vi "Intialise or refresh queue.vi"(2 "When did you stick it in?":dbl, 3 "Cell Settings Array":T2(array[cluster])=[{"Measure?"=TRUE, "Area (cm^2)"=0.0, "Cell Label"="", "Cell Description"="", "Time between scans (s)"=0.0, "Cell Position"=1, "Scan settings in queue"=0, "Sample holder"=4.0}, {"Measure?"=TRUE, "Area (cm^2)"=0.0, "Cell Label"="", "Cell Description"="", "Time between scans (s)"=0.0, "Cell Position"=2, "Scan settings in queue"=0, "Sample holder"=4.0}, {"Measure?"=TRUE, "Area (cm^2)"=0.0, "Cell Label"="", "Cell Description"="", "Time between scans (s)"=0.0, "Cell Position"=3, "Scan settings in queue"=0, "Sample holder"=4.0}, {"Measure?"=TRUE, "Area (cm^2)"=0.0, "Cell Label"="", "Cell Description"="", "Time between scans (s)"=0.0, "Cell Position"=4, "Scan settings in queue"=0, "Sample holder"=4.0}, {"Measure?"=TRUE, "Area (cm^2)"=0.0, "Cell Label"="", "Cell Description"="", "Time between scans (s)"=0.0, "Cell Position"=5, "Scan settings in queue"=0, "Sample holder"=4.0}, {"Measure?"=TRUE, "Area (cm^2)"=0.0, "Cell Label"="", "Cell Description"="", "Time between scans (s)"=0.0, "Cell Position"=6, "Scan settings in queue"=0, "Sample holder"=4.0}, {"Measure?"=TRUE, "Area (cm^2)"=0.0, "Cell Label"="", "Cell Description"="", "Time between scans (s)"=0.0, "Cell Position"=7, "Scan settings in queue"=0, "Sample holder"=4.0}, {"Measure?"=TRUE, "Area (cm^2)"=0.0, "Cell Label"="", "Cell Description"="", "Time between scans (s)"=0.0, "Cell Position"=8, "Scan settings in queue"=0, "Sample holder"=4.0}, {"Measure?"=TRUE, "Area (cm^2)"=0.0, "Cell Label"="", "Cell Description"="", "Time between scans (s)"=0.0, "Cell Position"=9, "Scan settings in queue"=0, "Sample holder"=4.0}, {"Measure?"=TRUE, "Area (cm^2)"=0.0, "Cell Label"="", "Cell Description"="", "Time between scans (s)"=0.0, "Cell Position"=10, "Scan settings in queue"=0, "Sample holder"=4.0}, {"Measure?"=TRUE, "Area (cm^2)"=0.0, "Cell Label"="", "Cell Description"="", "Time between scans (s)"=0.0, "Cell Position"=11, "Scan settings in queue"=0, "Sample holder"=4.0}, {"Measure?"=TRUE, "Area (cm^2)"=0.0, "Cell Label"="", "Cell Description"="", "Time between scans (s)"=0.0, "Cell Position"=12, "Scan settings in queue"=0, "Sample holder"=4.0}, {"Measure?"=TRUE, "Area (cm^2)"=0.0, "Cell Label"="", "Cell Description"="", "Time between scans (s)"=0.0, "Cell Position"=13, "Scan settings in queue"=0, "Sample holder"=4.0}, {"Measure?"=TRUE, "Area (cm^2)"=0.0, "Cell Label"="", "Cell Description"="", "Time between scans (s)"=0.0, "Cell Position"=14, "Scan settings in queue"=0, "Sample holder"=4.0}, {"Measure?"=TRUE, "Area (cm^2)"=0.0, "Cell Label"="", "Cell Description"="", "Time between scans (s)"=0.0, "Cell Position"=15, "Scan settings in queue"=0, "Sample holder"=4.0}, {"Measure?"=TRUE, "Area (cm^2)"=0.0, "Cell Label"="", "Cell Description"="", "Time between scans (s)"=0.0, "Cell Position"=16, "Scan settings in queue"=0, "Sample holder"=4.0}] {"Scan settings in queue" items=["Regular", "Inverted"]}, 4 "Queue in":T1(array[cluster]) {"Scan settings in queue" items=["Regular", "Inverted"]; "Time of the last scan (s)" format="%<%H:%M:%S>t"; "When did you stick it in?" format="%<%H:%M:%S>t"; "Time to next scan (s)" format="%<%H:%M:%S>t"; "Time in rig (s)" format="%<%H:%M:%S>t"}) -> (0 "Queue out":T1(array[cluster]) {"Scan settings in queue" items=["Regular", "Inverted"]; "Time of the last scan (s)" format="%<%H:%M:%S>t"; "When did you stick it in?" format="%<%H:%M:%S>t"; "Time to next scan (s)" format="%<%H:%M:%S>t"; "Time in rig (s)" format="%<%H:%M:%S>t"})   [LabVIEW 2011]
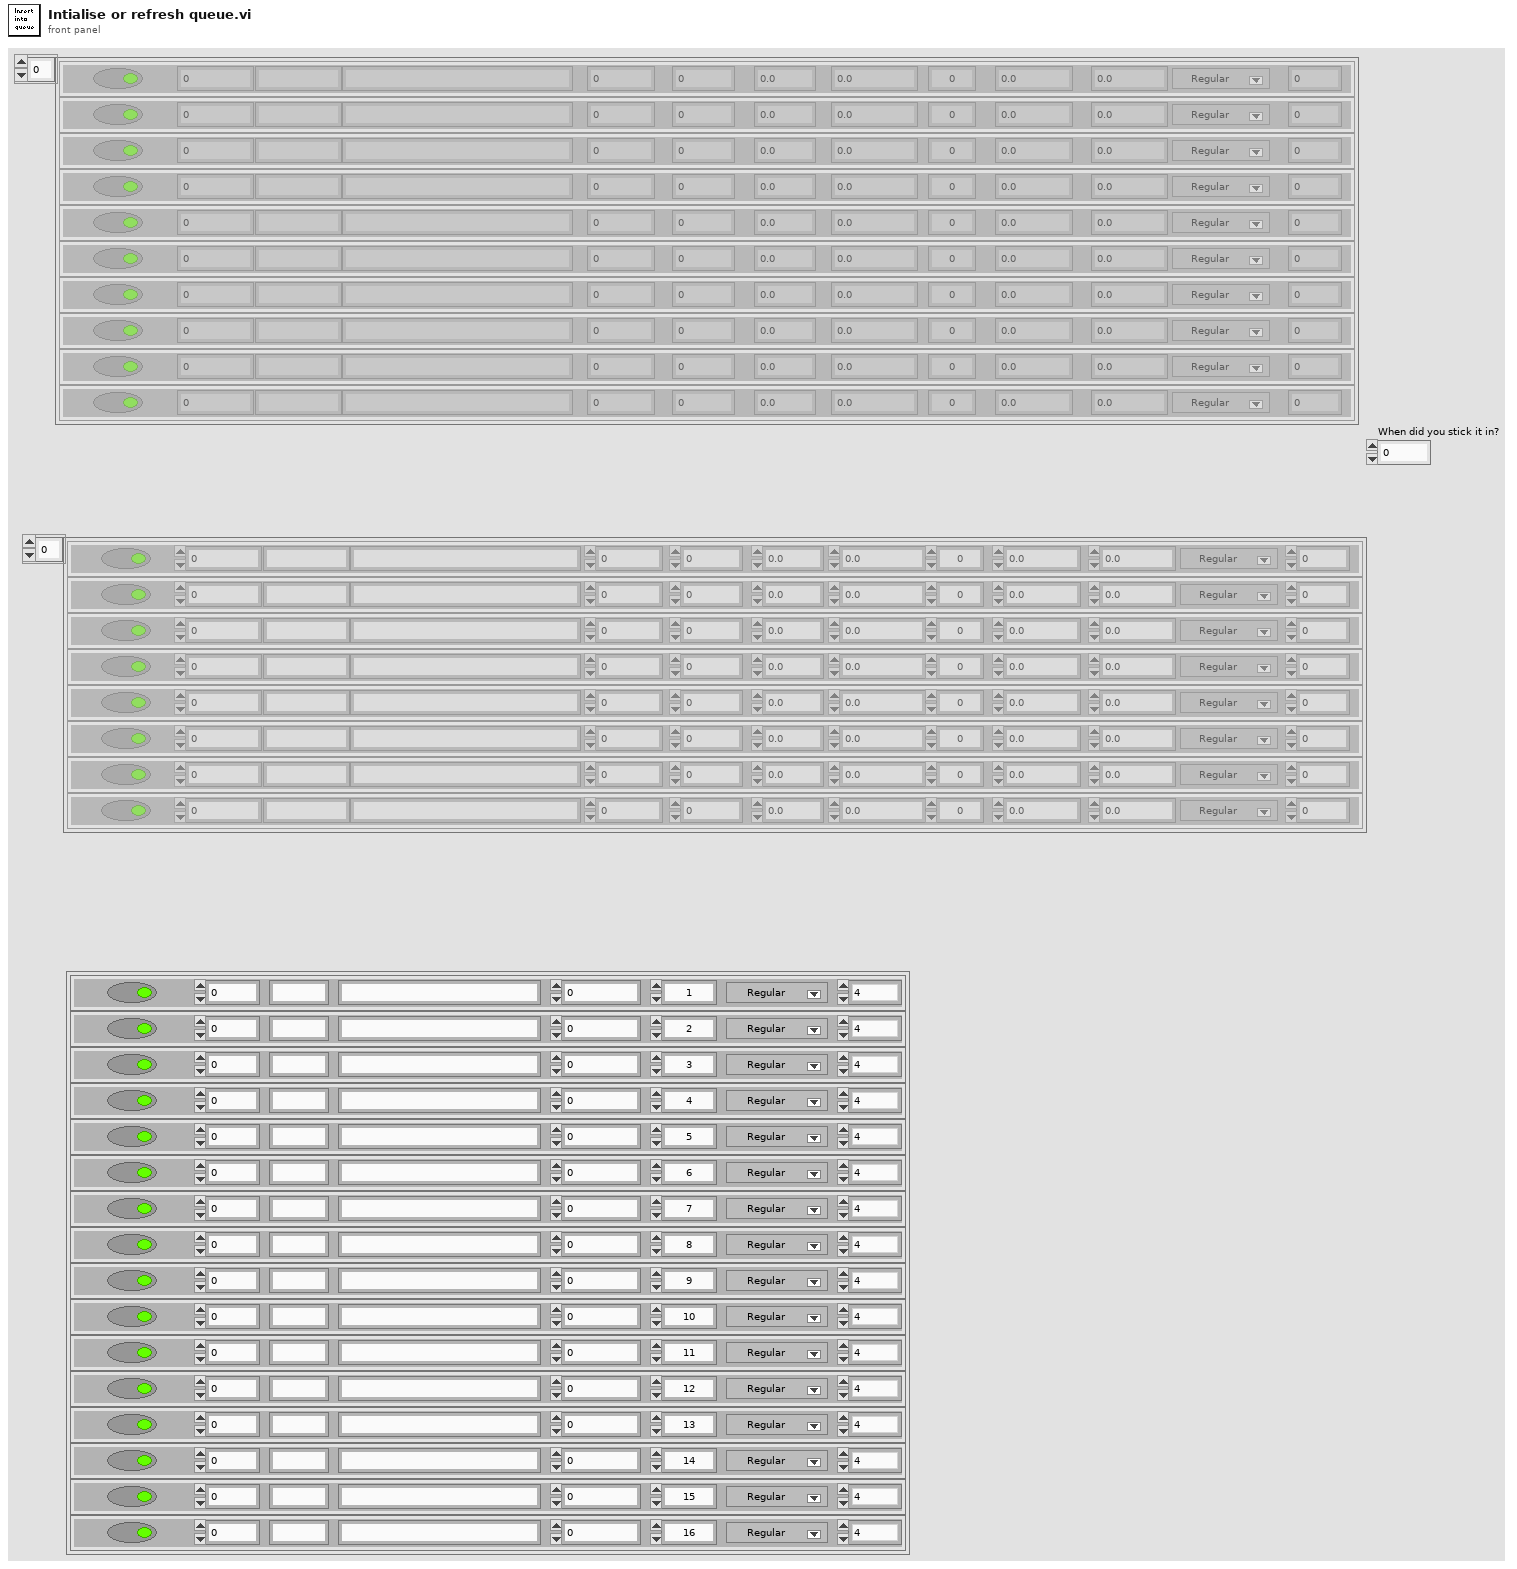
[diagram p1: front panel]
types:
  T1 = cluster{"Measure?":bool, "Area (cm^2)":dbl, "Cell Label":string, "Cell Description":string, "Cell Position":i32, "Time in rig (s)":dbl, "Time to next scan (s)":dbl, "Scan number":dbl, "When did you stick it in?":dbl, "Time between scans (s)":dbl, "Time of the last scan (s)":dbl, "Scan settings in queue":u16, "Sample Holder":dbl}[]
  T2 = cluster{"Measure?":bool, "Area (cm^2)":dbl, "Cell Label":string, "Cell Description":string, "Time between scans (s)":dbl, "Cell Position":i32, "Scan settings in queue":u16, "Sample holder":dbl}[]
  T3 = cluster{"Measure?":bool, "Area (cm^2)":dbl, "Cell Label":string, "Cell Description":string, "Cell Position":i32, "Time in rig (h)":dbl, "Time to next scan (min)":dbl, "Scan number":dbl, "When did you stick it in?":dbl, "Time between scans (min)":dbl, "Time of the last scan(min)":dbl, "Scan settings in queue":u16, "Sample Holder":dbl}[]
  T4 = cluster{"Measure?":bool, "Area (cm^2)":dbl, "Cell Label":string, "Cell Description":string, "Cell Position":i32, "Time in rig (s)":dbl, "Time to next scan (s)":dbl, "Scan number":dbl, "When did you stick it in?":dbl, "Time between scans (s)":dbl, "Time of the last scan (s)":dbl, "Scan settings in queue":u16, "Sample Holder":dbl}
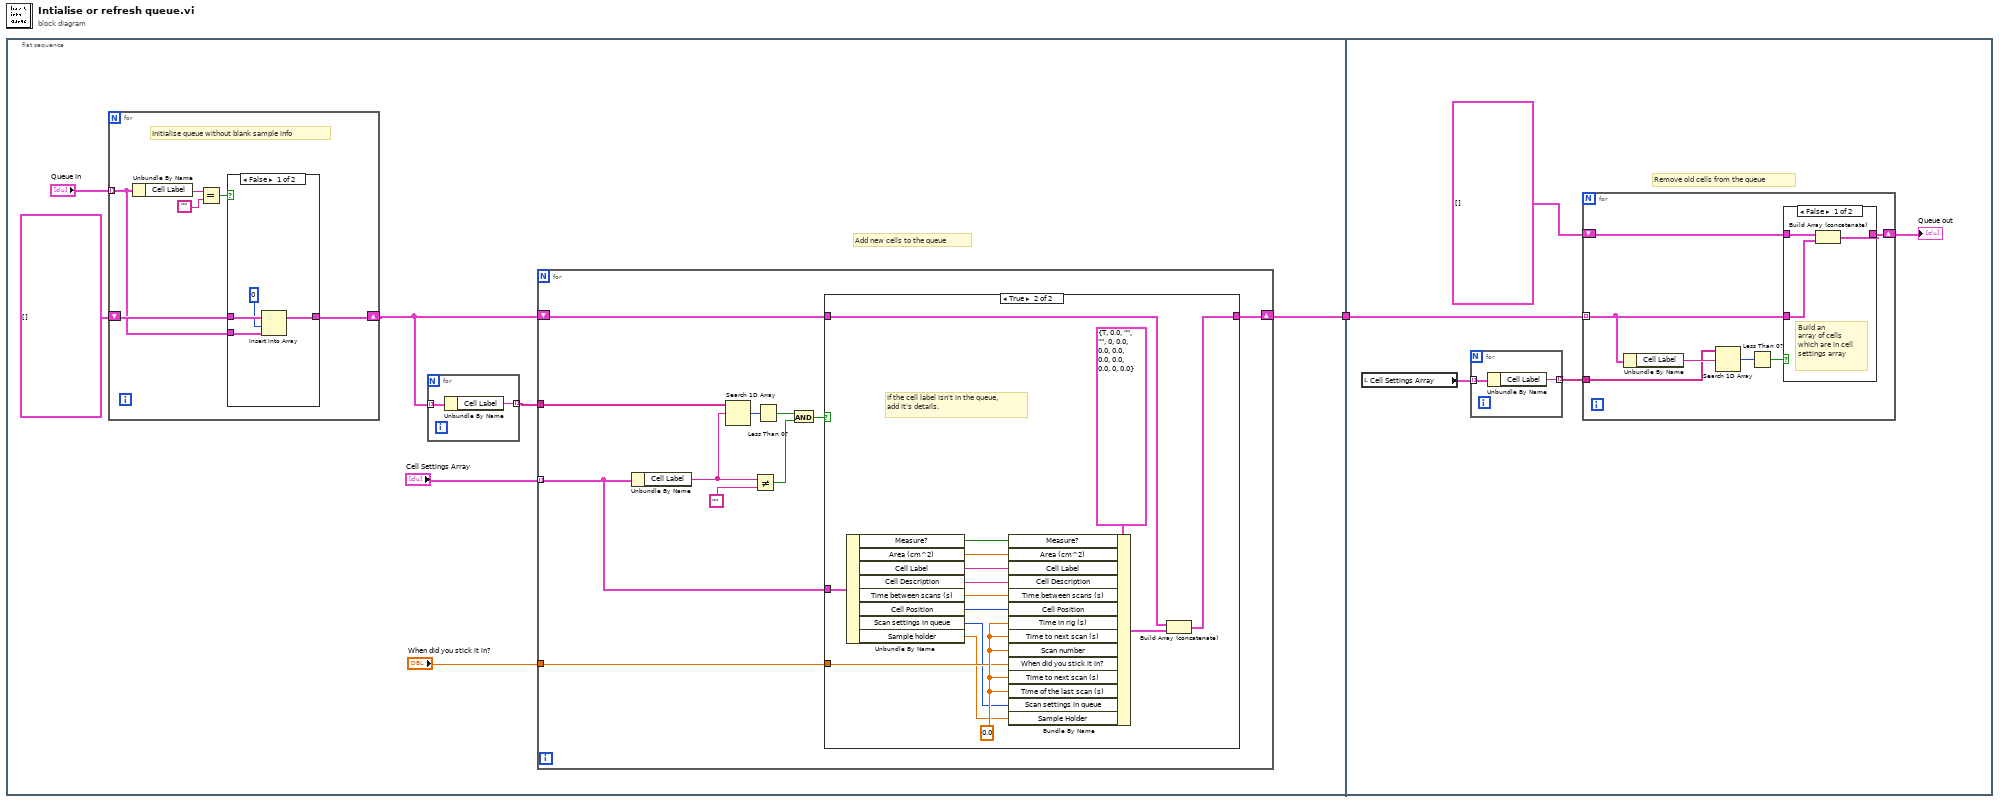
[diagram p0: block diagram]
diagram:
  n1 = flat-sequence {
    tunnel: [w3] -> w1
    tunnel: w1 -> [w49]
    frame #0 {
      # "Add new cells to the queue"
      n2 = for {
        tunnel: "Queue in" -> [w10] mode=indexing
        shift-right: [w9] -> w2
        shift-left: T3 [] -> [w11]
        # "Initialise queue without blank sample info"
        n3 = Unbundle By Name(w10) -> ("Cell Label"=w14:string)
        n4 = Equal?(x=w14, y="") -> (x = y?=w12:bool)
        n5 = case shown="False" w12 {
          tunnel: w11 -> [w18 w19]
          tunnel: w10 -> [w16 _]
          tunnel: [w15 w19] -> w9
          frame False {
            n6 = Insert Into Array(array=w18, index=0, new element=w16) -> (w15:T3)
          }
          frame True {
          }
        }
      }
      n7 = for {
        tunnel: w2 -> [w21] mode=indexing
        tunnel: [w20] -> w7 mode=indexing
        n8 = Unbundle By Name(w21) -> ("Cell Label"=w20:string)
      }
      n9 = for {
        tunnel: "Cell Settings Array" -> [w29] mode=indexing
        tunnel: "When did you stick it in?" -> [w30]
        tunnel: w7 -> [w31]
        shift-right: [w27] -> w3
        shift-left: w2 -> [w28]
        n10 = Unbundle By Name(w29) -> ("Cell Label"=w25:string)
        n11 = Search 1D Array(1D array=w31, element=w25) -> (index of element=w32:i32)  [unwired: 1 in]
        n12 = Not Equal?(x=w25, y="") -> (x != y?=w23:bool)
        n13 = Less Than 0?(x=w32) -> (x < 0?=w26:bool)
        n14 = And(x=w26, y=w23) -> (x .and. y?=w22:bool)
        n15 = case shown="True" w22 {
          tunnel: w30 -> [_ w46]
          tunnel: w29 -> [_ w45]
          tunnel: w28 -> [w33 w36]
          tunnel: [w33 w35] -> w27
          frame False {
          }
          frame True {
            w48 = 0.0 ("Time of the last scan (min)")
            # "If the cell label isn't in the queue,\nadd it's details."
            n16 = Unbundle By Name(w45) -> ("Measure?"=w44:bool, "Area (cm^2)"=w43:dbl, "Cell Label"=w42:string, "Cell Description"=w41:string, "Time between scans (s)"=w40:dbl, "Cell Position"=w39:i32, "Scan settings in queue"=w38:u16, "Sample holder"=w34:dbl)
            n17 = Bundle By Name(cluster=T4 {"Measure?"=TRUE, "Area (cm^2)"=0.0, "Cell Label"="", "Cell Description"="", "Cell Position"=0, "Time in rig (s)"=0.0, "Time to next scan (s)"=0.0, "Scan number"=0.0, "When did you stick it in?"=0.0, "Time between scans (s)"=0.0, "Time of the last scan (s)"=0.0, "Scan settings in queue"=0, "Sample Holder"=0.0} ("Cluster"), "Measure?"=w44, "Area (cm^2)"=w43, "Cell Label"=w42, "Cell Description"=w41, "Time between scans (s)"=w40, "Cell Position"=w39, "Time in rig (s)"=w48, "Time to next scan (s)"=w48, "Scan number"=w48, "When did you stick it in?"=w46, "Time to next scan (s)"=w48, "Time of the last scan (s)"=w48, "Scan settings in queue"=w38, "Sample Holder"=w34) -> (w37:T4)
            n18 = Build Array (concatenate)(w36, w37) -> (w35:T1)
          }
        }
      }
    }
    frame #1 {
      # "Remove old cells from the queue"
      n19 = local read "Cell Settings Array"() -> (w52:T2)
      n20 = for {
        tunnel: w52 -> [w55] mode=indexing
        tunnel: [w54] -> w50 mode=indexing
        n21 = Unbundle By Name(w55) -> ("Cell Label"=w54:string)
      }
      n22 = for {
        tunnel: w50 -> [w61]
        tunnel: w49 -> [w57] mode=indexing
        shift-right: [w56] -> w53
        shift-left: T3 [] -> [w59]
        n23 = Unbundle By Name(w57) -> ("Cell Label"=w62:string)
        n24 = Search 1D Array(1D array=w61, element=w62) -> (index of element=w60:i32)  [unwired: 1 in]
        n25 = Less Than 0?(x=w60) -> (x < 0?=w58:bool)
        n26 = case shown="False" w58 {
          tunnel: w59 -> [w65 w66]
          tunnel: w57 -> [w64 _]
          tunnel: [w63 w66] -> w56
          frame False {
            # "Build an\narray of cells\nwhich are in cell\nsettings array"
            n27 = Build Array (concatenate)(w65, w64) -> (w63:T3)
          }
          frame True {
          }
        }
      }
      "Queue out" <- w53
    }
  }
